vi "VL16.vi"() -> ()   [LabVIEW 2019]
uses:
  <vilib>/Math Plots/3D Math Plots/3D Contour/3D Contour XCtrl/3D Contour.xctl
  <vilib>/Math Plots/3D Math Plots/3D Contour/3D Contour Datatype/Public/Plot Helper (Matrix).vi
  <vilib>/Math Plots/3D Math Plots/3D Contour/3D Contour Datatype/3D Contour Datatype.lvclass
panel:
  out "size":i32
  out "Frames/Sec Processing":dbl=19.657052874295836 format="%#_2g"
  out "3D Contour":refnum<class "3D Plot Datatype.lvclass">[](xcontrol)
  in  "탭 컨트롤":enum32{"3D Display", "xy graph", "Data", "etc"}(tab)
  out "3D LIDAR Data":refnum<vi>(3d-picture)
  out "Frames/Sec display":dbl=19.657052874295836 format="%#_2g"
  out "XY Graph":cluster{sgl[], sgl[]}(graph)
  out "size(s)":i32
  out "size(s) 2":i32
  out "Data":T1(array[cluster])
  out "Array":cluster{"x":dbl, "y":dbl, "z":dbl}[](array[cluster])
  out "gridmap 3":dbl[][](array[numeric])
  out "Color Map":dbl[][](graph)
  out "색 테이블":u32[](array[numeric])
  in  "LiDAR Offset":T2 {"Z_Rotation[Deg]" format="%#.2f"; "Y_Rotation[Deg]" format="%#.2f"; "X_Rotation[Deg]" format="%#.2f"; "Z_offset[m]" format="%#.2f"; "Y_offset[m]" format="%#.2f"; "X_offset[m]" format="%#.2f"}
  out "In Range Data":T1(array[cluster])
  in  "Robot Status":T3
  in  "Initial Grid":dbl[][](array[numeric])
  out "obstacle2Out":dbl[][](array[numeric])
  in  "obstacle2":dbl[][](array[numeric])=[[1000.0], [1000.0]]
  in  "InitialGrid":cluster{"x":dbl, "y":dbl}[](array[cluster])
  in  "Index":dbl[][](array[numeric])
  in  "gridmap":dbl[][](array[numeric])=[[0.0, 0.0, 0.0, 0.0], [0.0, 0.0, 0.0, 0.0]]
  in  "stop":bool
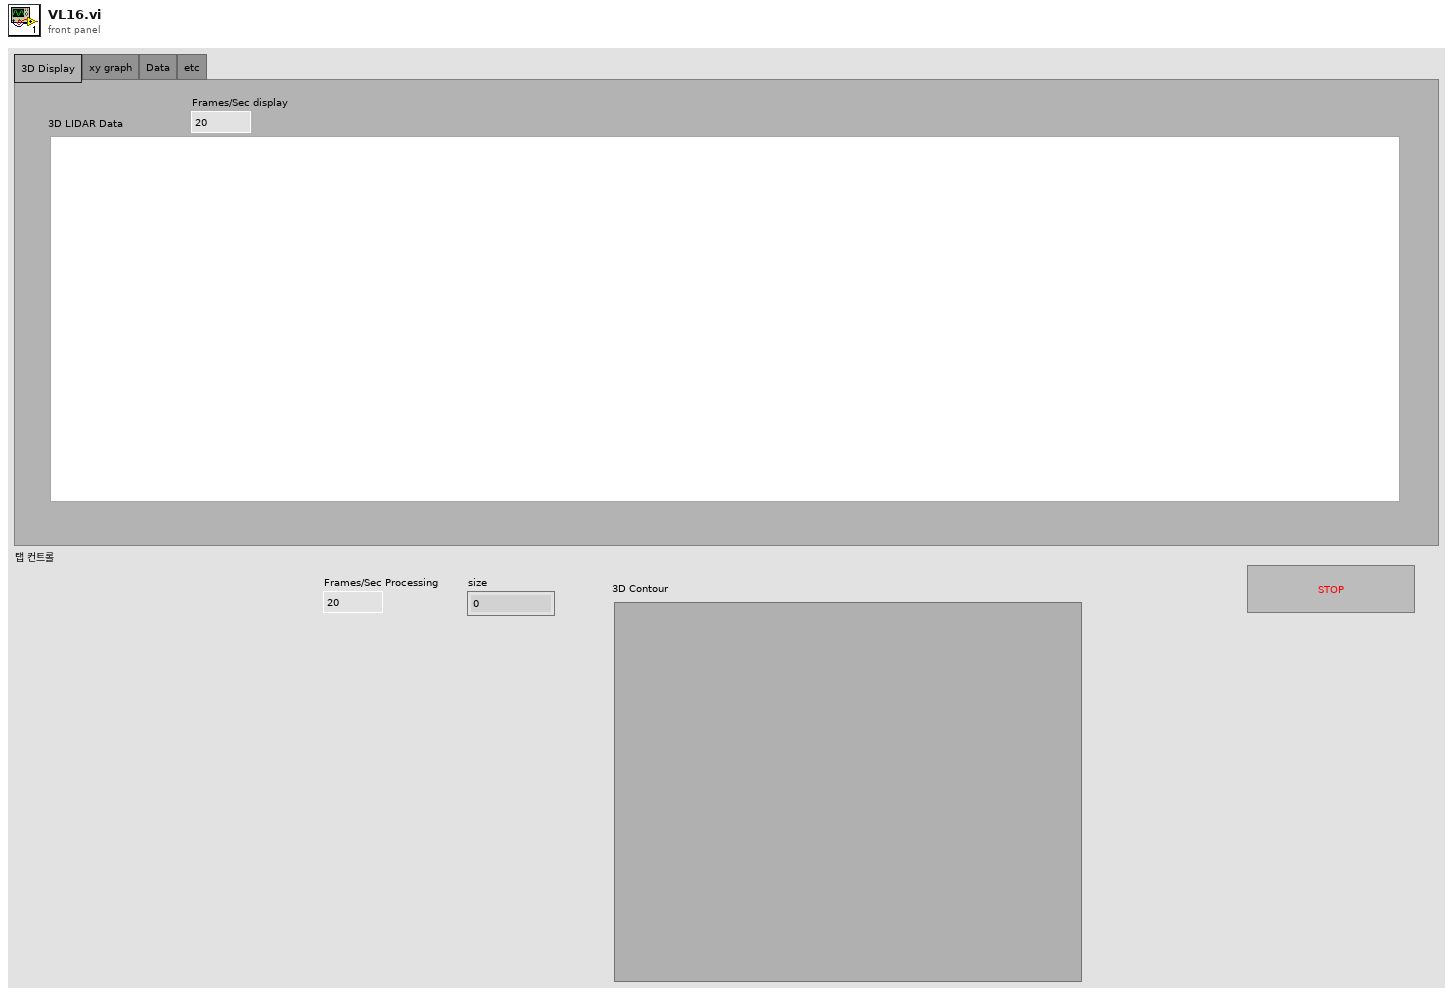
[diagram p1: front panel]
types:
  T1 = cluster{"id":i32, "arimuth(degree)":dbl, "vertical(degree)":dbl, "distance(meter)":dbl, "reflectivity":u8, "times(s)":ext, "x":dbl, "y":dbl, "z":dbl}[]
  T2 = cluster{"X_offset[m]":sgl, "Y_offset[m]":sgl, "Z_offset[m]":sgl, "X_Rotation[Deg]":sgl, "Y_Rotation[Deg]":sgl, "Z_Rotation[Deg]":sgl}
  T3 = cluster{"X (m)":dbl, "Y (m)":dbl, "Z (m)":dbl, "Roll (degree)":dbl, "Pitch (degree)":dbl, "Heading (degree)":dbl, "Linear velocity (m/s)":dbl, "Angular velocity (rad/s)":dbl}
  T4 = enum16{"Points", "Lines", "Line Strip", "Line Loop", "Triangles", "Triangle Strip", "Triangle Fan", "Quads", "Quad Strip", "Polygon"}
  T5 = enum16{"Overall", "Per Primitive", "Per Vertex", "Binding Off"}
  T6 = typedef "LVRGBAColorTypeDef.ctl" = cluster{"Red":sgl, "Green":sgl, "Blue":sgl, "Alpha":sgl}
  T7 = cluster{"id":i32, "azimuth(degree)":dbl, "vertical(degree)":dbl, "distance(meter)":dbl, "reflectivity":u8, "time(s)":ext, "x":dbl, "y":dbl, "z":dbl}
  T8 = cluster{"id":i32, "azimuth(degree)":dbl, "vertical(degree)":dbl, "distance(meter)":dbl, "reflectivity":u8, "time(s)":ext, "x":dbl, "y":dbl, "z":dbl}[]
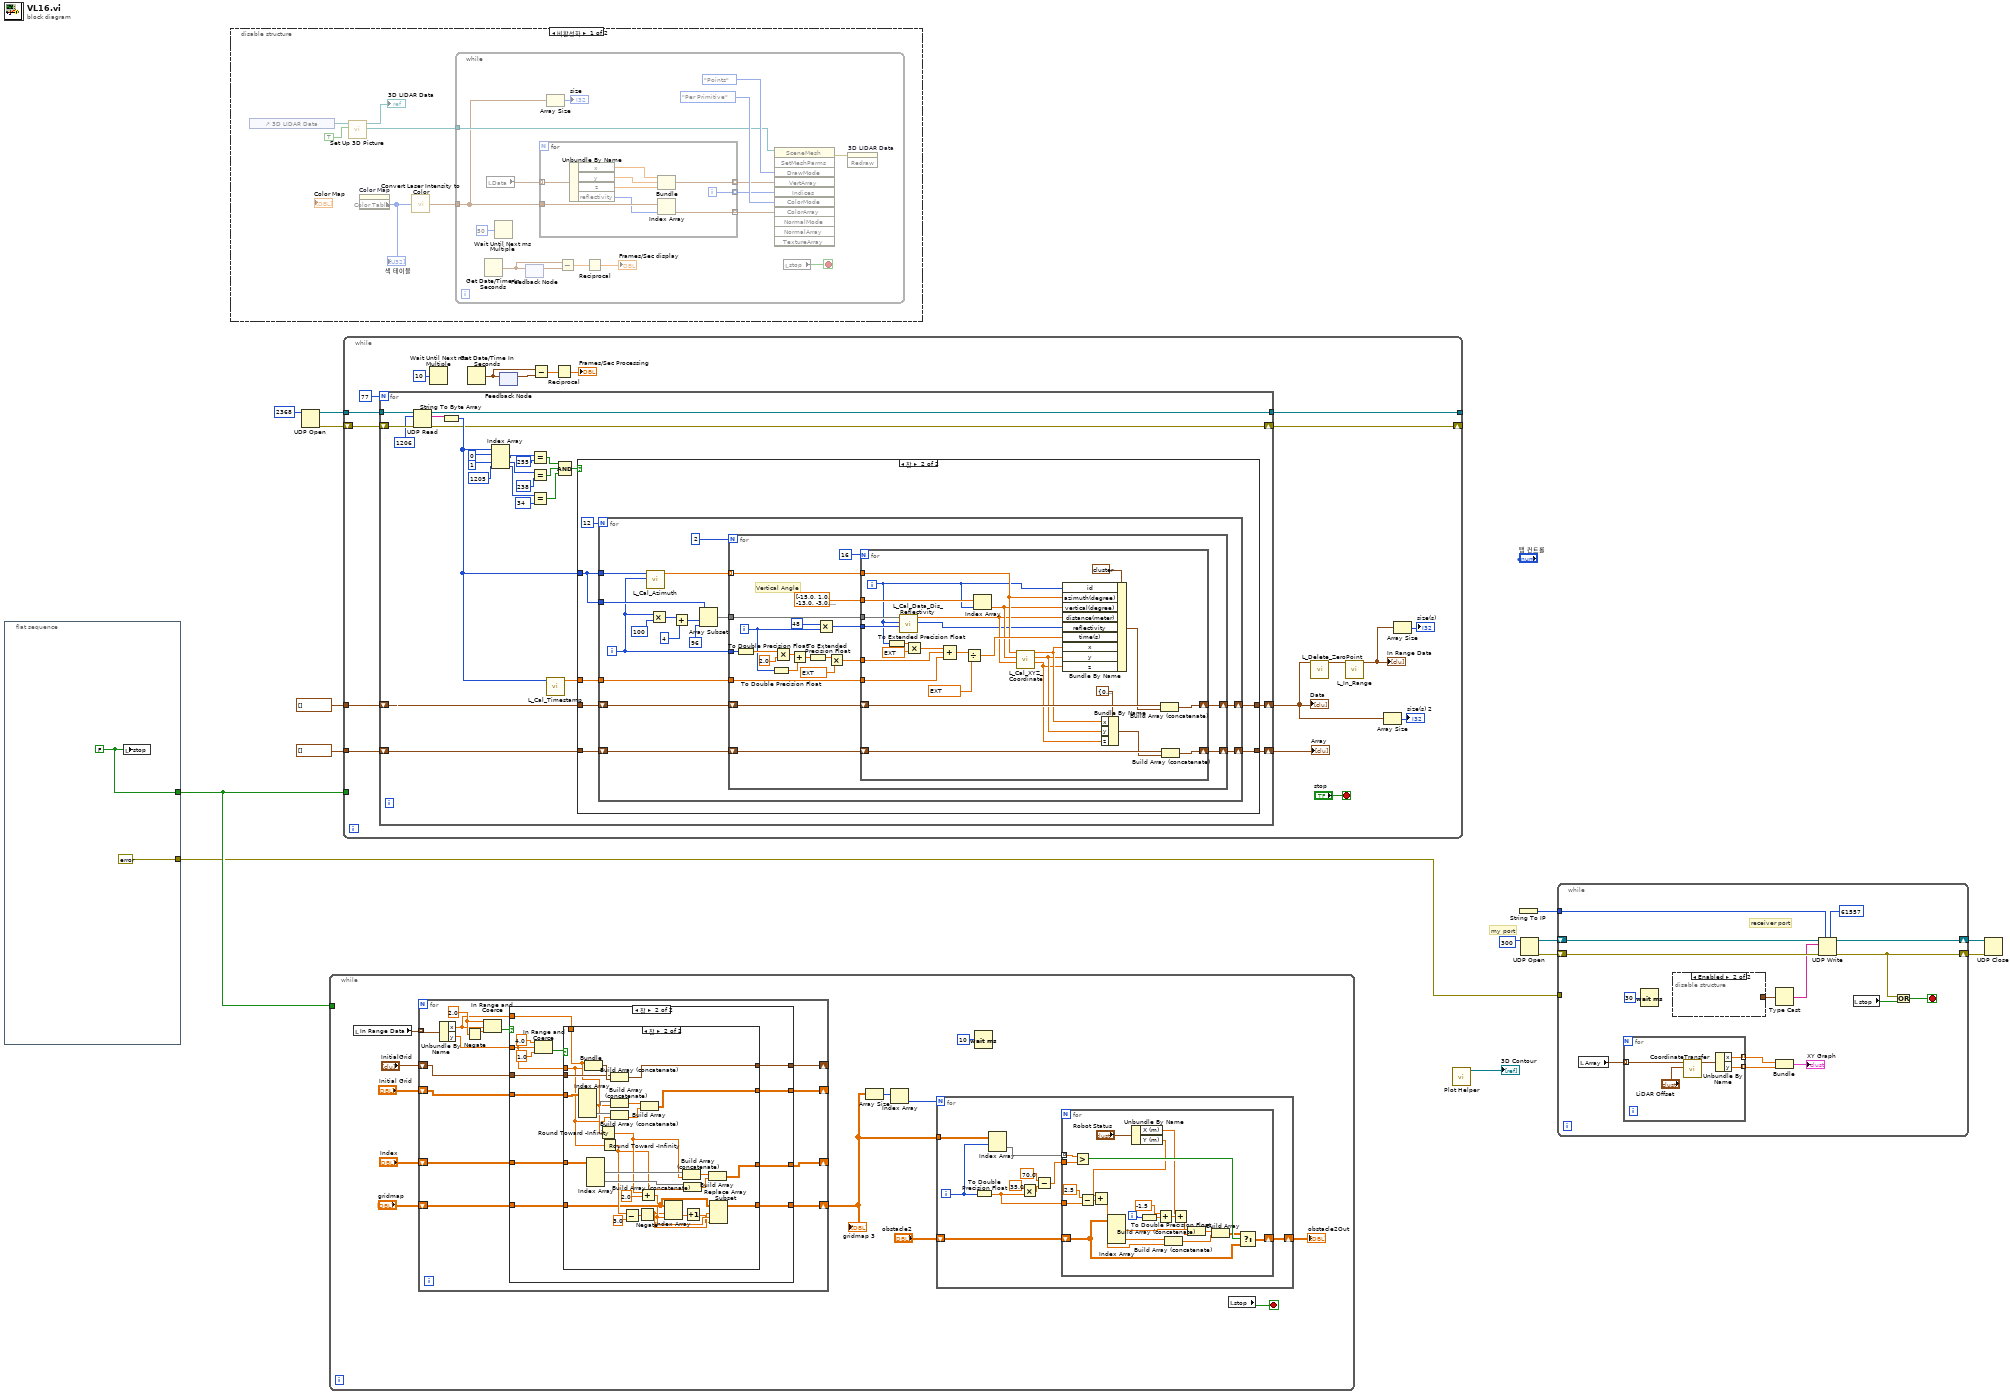
[diagram p0: block diagram]
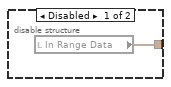
[diagram p5: hidden frame]
diagram:
  # "my port"
  n1 = flat-sequence {
    tunnel: [w16] -> w3
    tunnel: [errorcluster {"status"=FALSE, "code"=0, "source"=""} ("에러 상수")] -> w2
    frame #0 {
      w16 = FALSE ("stop")
      n2 = local write "stop"(w16) -> ()
    }
  }
  n3 = disable-structure shown="비활성화" {
    frame Disabled {
      n4 = control-ref of="3D LIDAR Data"() -> (w22:refnum<vi>)
      n5 = call <instrlib>:"Set Up 3D Picture.vi"("Reset Camera on Start"=TRUE, "3D Picture Control In"=w22) -> ("Mesh Out"=w19:refnum<vi>, "Scene Out"=→"3D LIDAR Data":refnum<vi>)  [unwired: 8 in]
      n6 = property on="Color Map" class="IntGraph (엄격한)"() -> ("Color Table"=w17:u32[])  [unwired: 2 in, 2 out]
      "색 테이블" <- w17
      n7 = call <instrlib>:"Convert Laser Intensity to Color.vi"("Color Table"=w17) -> ("Color Array"=w20:T6[])  [unwired: 8 in]
      n8 = while {
        tunnel: w19 -> [w26]
        tunnel: w20 -> [w23]
        stop <- w27 stop-if-true
        n9 = Get Date/Time In Seconds() -> (seconds since 1Jan1904=w38:timestamp)
        n10 = local read "Data"() -> (w24:T1)
        n11 = Wait Until Next ms Multiple(millisecond multiple=u32 50) -> ()  [unwired: 1 out]
        n12 = feedback #1() -> (w37:timestamp)  [unwired: 1 in]
        n13 = feedback-in #1(w38) -> ()
        n14 = for {
          tunnel: [w47] -> w31 mode=indexing
          tunnel: w23 -> [w46]
          tunnel: [w45] -> w29 mode=indexing
          tunnel: w24 -> [w44] mode=indexing
          tunnel: [w40] -> w30 mode=indexing
          i -> [w47]
          n15 = Unbundle By Name(w44) -> ("x"=w42:dbl, "y"=w41:dbl, "z"=w39:dbl, "reflectivity"=w43:u8)
          n16 = Bundle("x"=w42, "y"=w41, "z"=w39) -> (w40:cluster{"x":dbl, "y":dbl, "z":dbl})  [unwired: 1 in]
          n17 = Index Array(array=w46, index=w43) -> (element=w45:T6)
        }
        n18 = Array Size(array=w23) -> (size(s)=→"size":i32)
        n19 = Subtract(x=w38, y=w37) -> (x-y=w36:dbl)
        n20 = Reciprocal(x=w36) -> (1/x=→"Frames/Sec display":dbl)
        n21 = invoke class="SceneMesh" method="SetMeshParms"(reference=w26, "DrawMode"=T4."Points" ("Draw Mode"), "VertArray"=w30, "Indices"=w31, "ColorMode"=T5."Per Primitive" ("Color Binding Mode"), "ColorArray"=w29) -> (error out=w28:errorcluster)  [unwired: 5 in, 10 out]
        n22 = local read "stop"() -> (w27:bool)
        n23 = invoke on="3D LIDAR Data" class="SceneGraphDisp (strict)" method="Redraw"(error in=w28) -> ()  [unwired: 2 in, 3 out]
      }
    }
    frame Enabled {
    }
  }
  n24 = UDP Open(11:u16 2368 ("port")) -> (port=w12:refnum<k16>, 0:w11:errorcluster)  [unwired: 4 in, 1 out]
  n25 = while {
    tunnel: w3 -> [_]
    stop <- w54 stop-if-true
    n26 = local read "In Range Data"() -> (w55:T1)
    n27 = for {
      tunnel: w55 -> [w105] mode=indexing
      shift-right: [w98] -> _
      shift-left: "InitialGrid" -> [w99]
      shift-right: [w96] -> _
      shift-left: "Initial Grid" -> [w97]
      shift-right: [w94] -> _
      shift-left: "Index" -> [w95]
      shift-right: [w92] -> w50
      shift-left: "gridmap" -> [w93]
      w103 = 2.0
      n28 = Unbundle By Name(w105) -> ("x"=w100:dbl, "y"=w101:dbl)
      n29 = Negate(x=w103) -> (-x=w104:dbl)
      n30 = In Range and Coerce(upper limit=w103, x=w100, lower limit=w104) -> (In Range?=w102:bool)  [unwired: 1 out]
      n31 = case shown="참" w102 {
        tunnel: w101 -> [_ w119]
        tunnel: w100 -> [_ w118]
        tunnel: w99 -> [w109 w117]
        tunnel: [w109 w116] -> w98
        tunnel: w97 -> [w108 w115]
        tunnel: [w108 w114] -> w96
        tunnel: w95 -> [w107 w113]
        tunnel: [w107 w112] -> w94
        tunnel: w93 -> [w106 w111]
        tunnel: [w106 w110] -> w92
        frame False {
        }
        frame True {
          n32 = In Range and Coerce(upper limit=4.0, x=w119, lower limit=1.0) -> (In Range?=w120:bool)  [unwired: 1 out]
          n33 = case shown="참" w120 {
            tunnel: w119 -> [_ w144]
            tunnel: w118 -> [_ w145]
            tunnel: w117 -> [w126 w153]
            tunnel: [w126 w152] -> w116
            tunnel: w115 -> [w125 w151]
            tunnel: [w125 w146] -> w114
            tunnel: w113 -> [w124 w143]
            tunnel: [w124 w138] -> w112
            tunnel: w111 -> [w123 w131]
            tunnel: [w123 w127] -> w110
            frame False {
            }
            frame True {
              n34 = Index Array(array=w151) -> (element #1=w150:dbl[], element #2=w149:dbl[])  [unwired: 4 in]
              n35 = Bundle("x"=w145, "y"=w144) -> (w154:cluster{"x":dbl, "y":dbl})  [unwired: 1 in]
              n36 = Index Array(array=w143) -> (element #1=w142:dbl[], element #2=w141:dbl[])  [unwired: 4 in]
              n37 = Round Toward -Infinity(1:w145) -> (0:w137:dbl)
              n38 = Round Toward -Infinity(1:w144) -> (0:w135:dbl)
              n39 = Build Array (concatenate)(w153, w154) -> (w152:cluster{"x":dbl, "y":dbl}[])
              n40 = Build Array (concatenate)(w150, w145) -> (w148:dbl[])
              n41 = Build Array (concatenate)(w149, w144) -> (w147:dbl[])
              n42 = Subtract(x=w135, y=3.0) -> (x-y=w133:dbl)
              n43 = Negate(x=w133) -> (-x=w129:dbl)
              n44 = Add(x=w137, y=2.0) -> (x+y=w130:dbl)
              n45 = Build Array(w148, w147) -> (w146:dbl[][])
              n46 = Index Array(array=w131, index (row)=w129, index (col)=w130) -> (element=w132:dbl)
              n47 = Build Array (concatenate)(w142, w137) -> (w140:dbl[])
              n48 = Build Array (concatenate)(w141, w135) -> (w139:dbl[])
              n49 = Increment(x=w132) -> (x+1=w128:dbl)
              n50 = Build Array(w140, w139) -> (w138:dbl[][])
              n51 = Replace Array Subset(array=w131, new element=w128, index (row)=w129, index (col)=w130) -> (w127:dbl[][])
            }
          }
        }
      }
    }
    "gridmap 3" <- w50
    n52 = Array Size(array=w50) -> (size(s)=w53:i32[])
    n53 = Index Array(array=w53) -> (element=w48:i32)  [unwired: 1 in]
    n54 = for {
      N: w48 -> [_]
      tunnel: w50 -> [w68]
      shift-right: [w61] -> w51
      shift-left: "obstacle2" -> [w62]
      i -> [w66]
      n55 = To Double Precision Float(number=w66) -> (double precision float=w60:dbl)
      n56 = Index Array(array=w68, index (row)=w66) -> (element=w67:dbl[])  [unwired: 1 in]
      n57 = Multiply(x=35.0, y=w60) -> (x*y=w65:dbl)
      n58 = Subtract(x=70.0, y=w65) -> (x-y=w63:dbl)
      n59 = for {
        tunnel: w67 -> [w91] mode=indexing
        tunnel: w63 -> [w90]
        tunnel: w60 -> [w71]
        shift-right: [w79] -> w61
        shift-left: w62 -> [w80]
        i -> [w89]
        n60 = Greater?(x=w91, y=w90) -> (0:w82:bool)
        n61 = Subtract(x=2.5 ("y"), y=w71) -> (x-y=w72:dbl)
        n62 = Index Array(array=w80) -> (element #1=w86:dbl[], element #2=w85:dbl[])  [unwired: 4 in]
        n63 = Unbundle By Name("Robot Status") -> ("X (m)"=w76:dbl, "Y (m)"=w75:dbl)
        n64 = Add(x=w75, y=w72) -> (x+y=w74:dbl)
        n65 = To Double Precision Float(number=w89) -> (double precision float=w88:dbl)
        n66 = Add(x=-1.5, y=w88) -> (x+y=w78:dbl)
        n67 = Build Array (concatenate)(w85, w74) -> (w83:dbl[])
        n68 = Add(x=w76, y=w78) -> (x+y=w77:dbl)
        n69 = Build Array (concatenate)(w86, w77) -> (w84:dbl[])
        n70 = Build Array(w84, w83) -> (w81:dbl[][])
        n71 = Select(t=w81, s=w82, f=w80) -> (s? t:f=w79:dbl[][])
      }
    }
    "obstacle2Out" <- w51
    n72 = Wait (ms)(milliseconds to wait=u32 10 ("대기 시간 (ms)")) -> ()  [unwired: 1 out]
    n73 = local read "stop"() -> (w54:bool)
  }
  n74 = while {
    shift-right: [w171] -> _
    shift-left: w11 -> [w172]
    tunnel: T1 [] -> [w170]
    tunnel: w12 -> [w173]
    tunnel: [w167] -> _
    tunnel: cluster{"x":dbl, "y":dbl, "z":dbl}[] [] -> [w161]
    tunnel: w3 -> [_]
    stop <- "stop" stop-if-true
    n75 = for {
      N: 77 -> [_]
      shift-right: [w178] -> w171
      shift-left: w172 -> [w181]
      shift-right: [w185] -> w155
      shift-left: w170 -> [w184]
      tunnel: w173 -> [w182]
      tunnel: [w177] -> w167
      shift-right: [w174] -> w160
      shift-left: w161 -> [w175]
      n76 = UDP Read(connection ID=w182, max size (548)=1206, 8:w181) -> (data out=w180:string, error out=w178:errorcluster, 3:w177:refnum<k16>)  [unwired: 1 in, 2 out]
      n77 = String To Byte Array(string=w180) -> (unsigned byte array=w179:u8[])
      n78 = Index Array(array=w179, index #1=0 ("index"), index #2=1 ("index"), index #3=1205 ("index")) -> (element #1=w195:u8, element #2=w192:u8, element #3=w190:u8)
      n79 = Equal?(x=w195, y=u8 255) -> (x = y?=w189:bool)
      n80 = Equal?(x=w192, y=u8 238) -> (x = y?=w188:bool)
      n81 = Equal?(x=w190, y=u8 34) -> (x = y?=w187:bool)
      n82 = call "L_Cal_Timestamp.vi"("data"=w179) -> ("Timestamp"=w186:ext)  [unwired: 10 in]
      n83 = Compound Arithmetic op=AND(w189, w188, w187) -> (w183:bool)
      n84 = case shown="참" w183 {
        tunnel: w186 -> [_ w207]
        tunnel: w179 -> [_ w206]
        tunnel: [w200 w205] -> w185
        tunnel: w184 -> [w200 w204]
        tunnel: w175 -> [w199 w202]
        tunnel: [w199 w201] -> w174
        frame False {
        }
        frame True {
          n85 = for {
            N: 12 -> [_]
            tunnel: w206 -> [w223]
            tunnel: w207 -> [w212]
            tunnel: w206 -> [w217]
            shift-right: [w210] -> w205
            shift-left: w204 -> [w211]
            shift-right: [w208] -> w201
            shift-left: w202 -> [w209]
            i -> [w213]
            n86 = call "L_Cal_Azimuth.vi"("DataBlock(-1)"=w213, "data"=w223) -> ("Azimuth(0,1)"=w222:dbl[])  [unwired: 9 in]
            n87 = Multiply(x=w213, y=100) -> (x*y=w214:i32)
            n88 = Add(x=w214, y=4) -> (x+y=w219:i32)
            n89 = Array Subset(array=w217, index=w219, length=96 ("index")) -> (w216:u8[])
            n90 = for {
              N: 2 -> [_]
              tunnel: w222 -> [w233] mode=indexing
              tunnel: w216 -> [w244]
              tunnel: w213 -> [w229]
              tunnel: w212 -> [w235]
              shift-right: [w231] -> w210
              shift-left: w211 -> [w232]
              shift-right: [w224] -> w208
              shift-left: w209 -> [w225]
              i -> [w226]
              # "Vertical Angle"
              n91 = To Double Precision Float(number=w229) -> (double precision float=w228:dbl)
              n92 = To Double Precision Float(number=w226) -> (double precision float=w227:dbl)
              n93 = Multiply(x=w228, y=2.0) -> (x*y=w239:dbl)
              n94 = Add(x=w239, y=w227) -> (x+y=w240:dbl)
              n95 = To Extended Precision Float(1:w240) -> (0:w241:ext)
              n96 = Multiply(x=48, y=w226) -> (x*y=w242:i32)
              n97 = Multiply(x=w241, y=ext 55.296) -> (x*y=w236:ext)
              n98 = for {
                N: 16 -> [_]
                tunnel: w244 -> [w271]
                tunnel: w242 -> [w270]
                tunnel: w236 -> [w266]
                tunnel: w235 -> [w265]
                tunnel: dbl[] [-15.0, 1.0, -13.0, -3.0, -11.0, 5.0, -9.0, 7.0, -7.0, 9.0, -5.0, 11.0, -3.0, 13.0, -1.0, 15.0] -> [w261]
                tunnel: w233 -> [w259]
                shift-right: [w253] -> w231
                shift-left: w232 -> [w256]
                shift-right: [w248] -> w224
                shift-left: w225 -> [w250]
                i -> [w254]
                n99 = To Extended Precision Float(1:w254) -> (0:w269:ext)
                n100 = call "L_Cal_Data_Dis_Reflectivity.vi"("Index(0 or 1)"=w270, "ID"=w254, "data"=w271) -> ("reflectivity"=w255:u8, "Distance"=w257:dbl)  [unwired: 7 in]
                n101 = Multiply(x=w269, y=ext 2.304) -> (x*y=w267:ext)
                n102 = Compound Arithmetic op=ADD(w267, w266, w265) -> (w263:ext)
                n103 = Divide(x=w263, y=ext 1000000.0) -> (x/y=w260:ext)
                n104 = Index Array(array=w261, index=w254) -> (element=w258:dbl)
                n105 = call "L_Cal_XYZ_Coordinate.vi"("distance"=w257, "vertical"=w258, "azimuth"=w259) -> ("z"=w245:dbl, "y"=w246:dbl, "x"=w247:dbl)  [unwired: 6 in]
                n106 = Bundle By Name(cluster=T7 {"id"=0, "azimuth(degree)"=0.0, "vertical(degree)"=0.0, "distance(meter)"=0.0, "reflectivity"=0, "time(s)"=0.0, "x"=0.0, "y"=0.0, "z"=0.0}, "id"=w254, "azimuth(degree)"=w259, "vertical(degree)"=w258, "distance(meter)"=w257, "reflectivity"=w255, "time(s)"=w260, "x"=w247, "y"=w246, "z"=w245) -> (w252:T7)
                n107 = Bundle By Name(cluster=cluster{"x":dbl, "y":dbl, "z":dbl} {"x"=0.0, "y"=0.0, "z"=0.0}, "x"=w247, "y"=w246, "z"=w245) -> (w249:cluster{"x":dbl, "y":dbl, "z":dbl})
                n108 = Build Array (concatenate)(w256, w252) -> (w253:T8)
                n109 = Build Array (concatenate)(w250, w249) -> (w248:cluster{"x":dbl, "y":dbl, "z":dbl}[])
              }
            }
          }
        }
      }
    }
    "Data" <- w155
    "Array" <- w160
    n110 = Wait Until Next ms Multiple(millisecond multiple=u32 10) -> ()  [unwired: 1 out]
    n111 = Get Date/Time In Seconds() -> (seconds since 1Jan1904=w165:timestamp)
    n112 = feedback #2() -> (w164:timestamp)  [unwired: 1 in]
    n113 = feedback-in #2(w165) -> ()
    n114 = Subtract(x=w165, y=w164) -> (x-y=w163:dbl)
    n115 = Reciprocal(x=w163) -> (1/x=→"Frames/Sec Processing":dbl)
    n116 = call "L_Delete_ZeroPoint.vi"("Data in"=w155) -> ("Data out"=w159:T1)  [unwired: 10 in]
    n117 = call "L_In_Range.vi"("Data"=w159) -> ("Data"=w158:T1)  [unwired: 14 in]
    "In Range Data" <- w158
    n118 = Array Size(array=w155) -> (size(s)=→"size(s) 2":i32)
    n119 = Array Size(array=w158) -> (size(s)=→"size(s)":i32)
  }
  n120 = call-poly <vilib>:"Plot Helper.vi"() -> ("3D Plot lvclass Array out"=→"3D Contour":refnum<class "3D Plot Datatype.lvclass">[])  [unwired: 6 in, 5 out]
  n121 = String To IP() -> (0:w6:u32)  [unwired: 1 in]
  n122 = UDP Open(11:u16 300 ("port")) -> (port=w5:refnum<k16>, 0:w4:errorcluster)  [unwired: 4 in, 1 out]
  n123 = while {
    tunnel: w6 -> [w283]
    shift-right: [w285] -> w8
    shift-left: w5 -> [w286]
    shift-right: [w281] -> w7
    shift-left: w4 -> [w284]
    tunnel: w2 -> [_]
    stop <- w282 stop-if-true
    # "receiver port"
    n124 = local read "Array"() -> (w272:cluster{"x":dbl, "y":dbl, "z":dbl}[])
    n125 = for {
      tunnel: [w291] -> w275 mode=indexing
      tunnel: [w290] -> w274 mode=indexing
      tunnel: w272 -> [w289] mode=indexing
      n126 = call "CoordinateTransfer.vi"("LiDAR Offset"="LiDAR Offset", "LiDAR Input"=w289) -> ("LiDAR Output"=w288:cluster{"x":sgl, "y":sgl, "z":sgl})  [unwired: 9 in]
      n127 = Unbundle By Name(w288) -> ("x"=w291:sgl, "y"=w290:sgl)
    }
    n128 = Wait (ms)(milliseconds to wait=u32 30) -> ()  [unwired: 1 out]
    n129 = disable-structure shown="Enabled" {
      disable-tunnel: [w292 _] -> w276
      frame Disabled {
        n130 = local read "In Range Data"() -> (w292:T1)
      }
      frame Enabled {
      }
    }
    n131 = Bundle(w275, w274) -> (→"XY Graph":cluster{sgl[], sgl[]})  [unwired: 1 in]
    n132 = Type Cast(x=w276) -> (*(type *) &x=w277:string)  [unwired: 1 in]
    n133 = UDP Write(address=w283, port or service name=u16 61557, connection ID=w286, data in=w277, 8:w284) -> (error out=w281:errorcluster, 3:w285:refnum<k16>)  [unwired: 1 in]
    n134 = local read "stop"() -> (w279:bool)
    n135 = Or(x=w281, y=w279) -> (x .or. y?=w282:bool)
  }
  n136 = UDP Close(connection ID=w8, 8:w7) -> ()  [unwired: 2 out]
